vi "In Range Speaker Left Limits.vi"(10 "offsetAngle V":dbl, 11 "offsetAngle H":dbl) -> (3 "Boolean":bool)   [LabVIEW 2023]
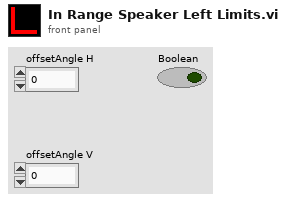
[diagram p1: front panel]
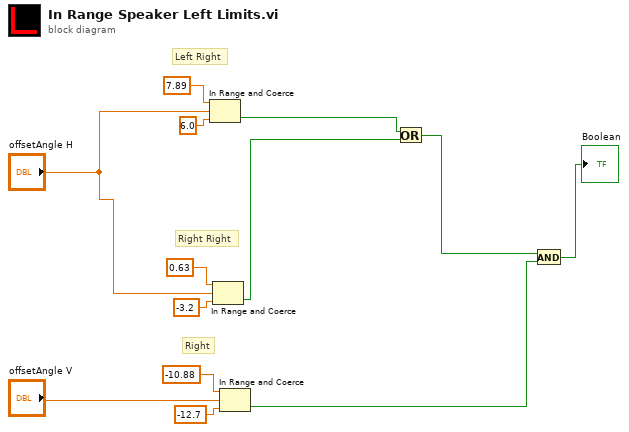
[diagram p0: block diagram]
diagram:
  # "Right"
  # "Right Right"
  # "Left Right"
  n1 = In Range and Coerce(upper limit=7.89, x="offsetAngle H", lower limit=6.0) -> (In Range?=w6:bool)  [unwired: 1 out]
  n2 = In Range and Coerce(upper limit=0.63, x="offsetAngle H", lower limit=-3.2) -> (In Range?=w2:bool)  [unwired: 1 out]
  n3 = In Range and Coerce(upper limit=-10.88, x="offsetAngle V", lower limit=-12.7) -> (In Range?=w1:bool)  [unwired: 1 out]
  n4 = Or(x=w6, y=w2) -> (x .or. y?=w3:bool)
  n5 = And(x=w3, y=w1) -> (x .and. y?=→"Boolean":bool)
